vi "NI9623_SUB-VI_ProvaDRV.vi"() -> ()   [LabVIEW 2020]
uses:
  TYPEDEF/NI9263_TD_Method.ctl
panel:
  in  "Numeric":dbl
  out "error out":errorcluster
  in  "Channels NI9263":tag="Dev1/ao0"
  in  "error in (no error)":errorcluster
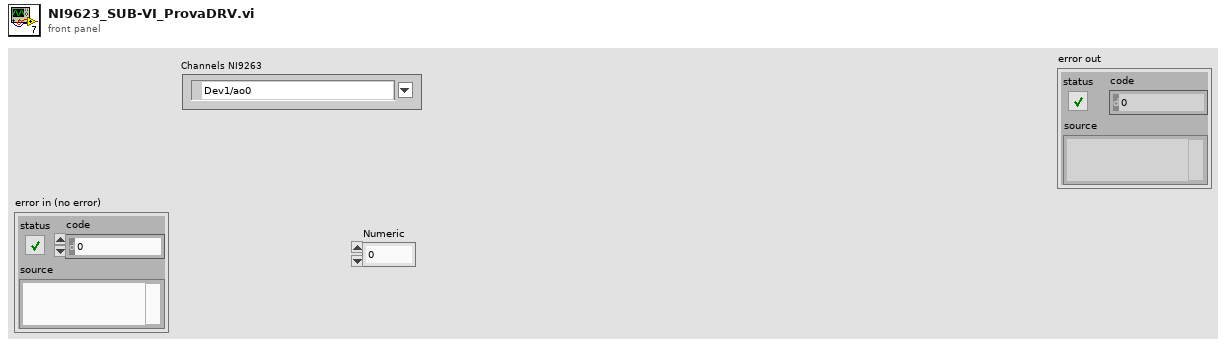
[diagram p1: front panel]
types:
  T1 = typedef "NI9263_TD_Method.ctl" = enum16{"NO_OP", "INIT", "SET", "GET", "CLOSE"}
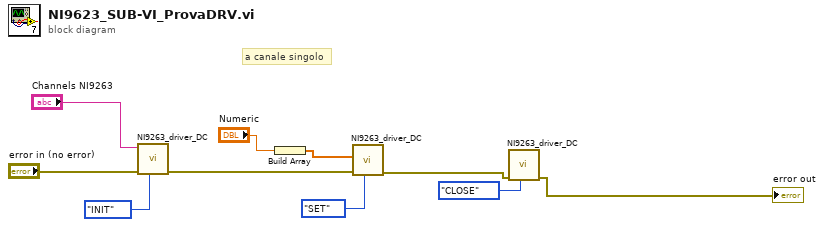
[diagram p0: block diagram]
diagram:
  # "a canale singolo"
  n1 = call "NI9263_driver_DC.vi"("METHOD"=NI9263_TD_Method."INIT", "error in (no error)"="error in (no error)", "Channels NI9263"="Channels NI9263") -> ("error out"=w7:errorcluster)  [unwired: 8 in]
  n2 = Build Array("Numeric") -> (w1:dbl[])
  n3 = call "NI9263_driver_DC.vi"("METHOD"=NI9263_TD_Method."SET", "error in (no error)"=w7, "Channel Values"=w1) -> ("error out"=w4:errorcluster)  [unwired: 8 in]
  n4 = call "NI9263_driver_DC.vi"("METHOD"=NI9263_TD_Method."CLOSE", "error in (no error)"=w4) -> ("error out"=→"error out":errorcluster)  [unwired: 9 in]
